vi "Cheap Encoder Read.vi"() -> (0 "Encoder Position":dbl format="%.3f")   [LabVIEW 2010]
uses:
  TMC Global.vi
panel:
  out "Error":bool
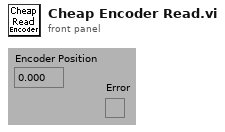
[diagram p1: front panel]
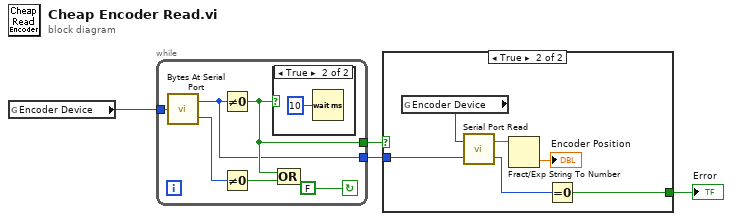
[diagram p0: block diagram]
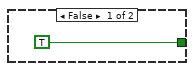
[diagram p3: hidden frame]
diagram:
  n1 = global read "TMC Global.vi" "Encoder Device"() -> (w4:i32)
  n2 = while {
    tunnel: [w7] -> w2
    tunnel: [w8] -> w3
    tunnel: w4 -> [w10]
    stop <- FALSE continue-if-true
    n3 = call <vilib>:"Bytes At Serial Port.vi"("port number"=w10) -> ("byte count"=w7:u32, "error code"=w6:i32)
    n4 = Not Equal To 0?(x=w7) -> (x != 0?=w8:bool)
    n5 = Not Equal To 0?(x=w6) -> (x != 0?=w9:bool)
    n6 = case shown="True" w8 {
      frame False {
      }
      frame True {
        n7 = Wait (ms)(milliseconds to wait=u32 10) -> ()  [unwired: 1 out]
      }
    }
    n8 = Compound Arithmetic op=OR(w8, w9) -> ()  [unwired: 1 out]
  }
  n9 = case shown="True" w3 {
    tunnel: w2 -> [_ w18]
    tunnel: [TRUE w13] -> w1
    frame False {
    }
    frame True {
      n10 = global read "TMC Global.vi" "Encoder Device"() -> (w17:i32)
      n11 = call <vilib>:"Serial Port Read.vi"("requested byte count"=w18, "port number"=w17) -> ("error code"=w14:i32, "string read"=w16:string)
      n12 = Fract/Exp String To Number(string=w16) -> (number=→"Encoder Position":dbl)  [unwired: 3 in, 1 out]
      n13 = Equal To 0?(x=w14) -> (x = 0?=w13:bool)
    }
  }
  "Error" <- w1
